vi "single_servo.vi"(2 "base_set":i32=-1, 3 "arm_set":i32=-1, 4 "ServoControl":enum16{"STOP", "both", "arm", "base"}(ring)) -> (1 "cmd":string)   [LabVIEW 2013]
uses:
  servo define.vi
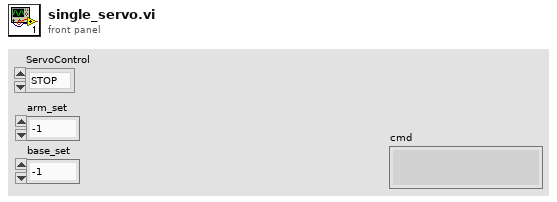
[diagram p1: front panel]
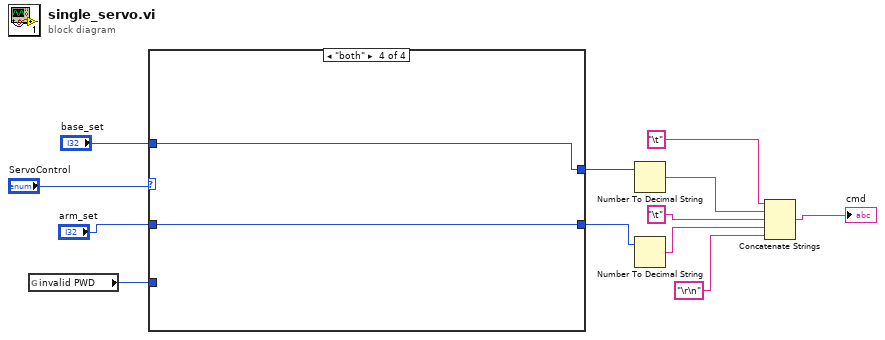
[diagram p0: block diagram]
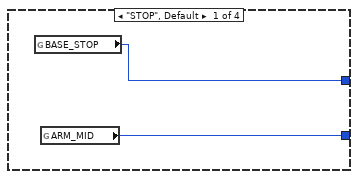
[diagram p2: hidden frame]
diagram:
  n1 = global read "servo define.vi" "invalid PWD"() -> (w1:i32)
  n2 = case shown="\"both\"" "ServoControl" {
    tunnel: [w14 w15 w18 w19] -> w10
    tunnel: [w13 w16 w17 w20] -> w9
    tunnel: "arm_set" -> [_ w16 _ w20]
    tunnel: "base_set" -> [_ _ w18 w19]
    tunnel: w1 -> [_ w15 w17 _]
    frame "STOP", Default {
      n3 = global read "servo define.vi" "BASE_STOP"() -> (w14:i32)
      n4 = global read "servo define.vi" "ARM_MID"() -> (w13:i32)
    }
    frame "arm" {
    }
    frame "base" {
    }
    frame "both" {
    }
  }
  n5 = Number To Decimal String(number=w10) -> (decimal integer string=w7:string)  [unwired: 1 in]
  n6 = Number To Decimal String(number=w9) -> (decimal integer string=w5:string)  [unwired: 1 in]
  n7 = Concatenate Strings("\t" ("ctr_buffer"), w7, "\t" ("ctr_buffer"), w5, "\r\n" ("ctr_buffer")) -> (→"cmd":string)
